vi "Sinusoidal Fit Display.vi"(11 "Positive Fit":refnum<class "Sinusoidal Fit.lvclass">) -> ()   [LabVIEW 2013]
uses:
  Typedef - Gain and Phase.ctl
  core/Classes/Sinusoidal Fit/Sinusoidal Fit.lvclass
  Typedef - Sinusoidal Fit Coefficients.ctl
panel:
  out "Stimulus":T1 {"Freq" format="%#.2f"; "Offset" format="%.3f"; "Gain" format="%.2f"; "Phase" format="%.1f"}
  out "Response":T1 {"Freq" format="%#.2f"; "Offset" format="%.3f"; "Gain" format="%.2f"; "Phase" format="%.1f"}
  out "Gain and Phase":T2 {"Phase SD" format="%.1f"; "Phase" format="%.1f"; "Gain SD" format="%.2f"; "Gain" format="%.2f"}
  # "Gain:"
  # "+/-"
  # "Phase:"
  # "+/-"
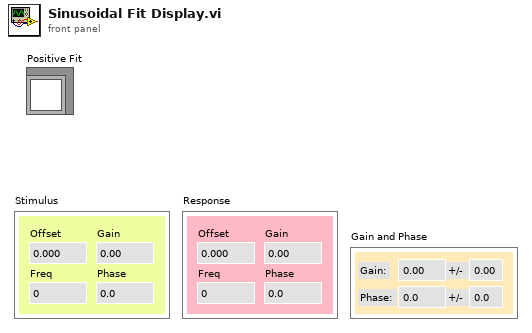
[diagram p1: front panel]
types:
  T1 = typedef "Typedef - Sinusoidal Fit Coefficients.ctl" = cluster{"Offset":dbl, "Gain":dbl, "Phase":dbl, "Freq":dbl}
  T2 = typedef "Typedef - Gain and Phase.ctl" = cluster{"Gain":dbl, "Gain SD":dbl, "Phase":dbl, "Phase SD":dbl}
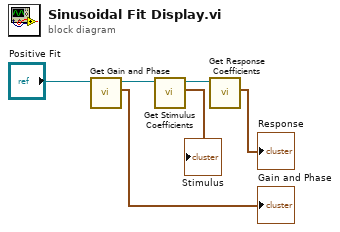
[diagram p0: block diagram]
diagram:
  n1 = call-dynamic "Get Gain and Phase.vi"("Sinusoidal Fit in"="Positive Fit") -> ("Gain and Phase"=→"Gain and Phase":T2, "Sinusoidal Fit out"=w5:refnum<class "Sinusoidal Fit.lvclass">)  [unwired: 8 in, 1 out]
  n2 = call-dynamic "Get Stimulus Coefficients.vi"("Sinusoidal Fit in"=w5) -> ("Coefficients"=→"Stimulus":T1, "Sinusoidal Fit out"=w4:refnum<class "Sinusoidal Fit.lvclass">)  [unwired: 8 in, 1 out]
  n3 = call-dynamic "Get Response Coefficients.vi"("Sinusoidal Fit in"=w4) -> ("Coefficients"=→"Response":T1)  [unwired: 8 in, 2 out]
